vi "LS M81_Suslov.vi"(1 "Action":T6=enum."Identify", 2 "Parameters":variant) -> (6 "Output":variant, 7 "Stop":bool)   [LabVIEW 2021]
uses:
  Sub Controls/Instrument Actions.ctl
  Sub Controls/Public.ctl
  Sub Controls/Instrument Match.ctl
  SubVIs/M81 Sensor Options.ctl
  Sub Controls/Factory Reset.ctl
  Sub Controls/Scan Output.ctl
  Sub Controls/Instrument IDN.ctl
  Sub Controls/User Event Command.ctl
  <vilib>/Instr/_visa.llb/VISA GPIB Control REN Mode.ctl
panel:
  in  "DC_AC Measurements":enum32{"DC", "Total RMS", "AC Peak-to-Peak"}(radio)
  out "Instrument Name":string
  in  "Source Mode":T1(radio)=enum."DC"
  in  "Sensor Mode":enum32{"No Selection", "DC", "AC", "Lockin"}(radio)=enum."DC"
  in  "Slot #":enum32{"Slot 1", "Slot 2", "Slot 3"}(radio)
  in  "Source Parameters":enum32{"DC Offset", "Peak-to-Peak/2", "Both"}(radio)=enum."Peak-to-Peak/2"
  in  "Factory Reset":T2
  out "Channel Index":i32
  in  "Lockin Measurements: RMS":T3={"X"=TRUE, "X&Y"=FALSE, "R"=FALSE, "R & ϴ"=FALSE}
  out "Title":string="Lake Shore M-81 Modules"
  in  "VISA resource name":refnum<visa-resource-name>
  in  "Instruments":T4[](array[typedef])=[{"Model"="VS-10", "Manufacturer"="Lake Shore", "Term Character"="", "Wait Time (mS)"=0, "Wait for SRQ"=FALSE, "Type"=""}, {"Model"="BCS-10", "Manufacturer"="Lake Shore", "Term Character"="", "Wait Time (mS)"=0, "Wait for SRQ"=FALSE, "Type"=""}, {"Model"="VM-10", "Manufacturer"="Lake Shore", "Term Character"="", "Wait Time (mS)"=0, "Wait for SRQ"=FALSE, "Type"=""}, {"Model"="CM-10", "Manufacturer"="Lake Shore", "Term Character"="", "Wait Time (mS)"=0, "Wait for SRQ"=FALSE, "Type"=""}]
  out "Model":string
  in  "Address":u16(ring)
  in  "Public":T5
  out "Measurement":dbl[](array[numeric]) format="%^.3e"
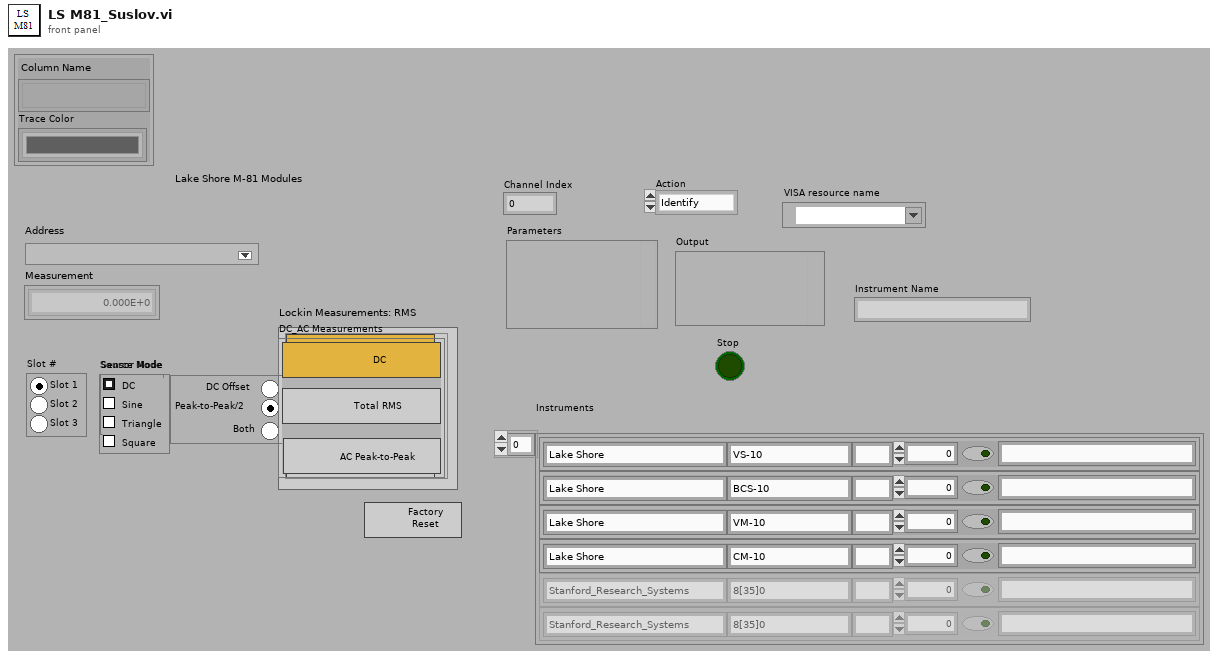
[diagram p1: front panel]
types:
  T1 = enum32{"No Selection", "DC", "Sine", "Triangle", "Square"}
  T2 = typedef "Factory Reset.ctl" = bool
  T3 = typedef "M81 Sensor Options.ctl" = cluster{"X":bool, "X&Y":bool, "R":bool, "R & ϴ":bool}
  T4 = typedef "Instrument Match.ctl" = cluster{"Model":string, "Manufacturer":string, "Term Character":string, "Wait Time (mS)":u32, "Wait for SRQ":bool, "Type":string}
  T5 = typedef "Public.ctl" = cluster{"Column Name":string[], "Trace Color":u32[]}
  T6 = typedef "Instrument Actions.ctl" = enum16{"Scan", "Identify", "New", "Configure", "Initialize", "Test", "Read", "Close"}
  T7 = typedef "Scan Output.ctl" = cluster{"Manufacturer":string, "Model":string, "Info":string, "Revision":string, "error out":errorcluster}
  T8 = typedef "Instrument IDN.ctl" = cluster{"VISA Address":string, "Status":u16, "Manufacturer":string, "Model":string, "Info":string, "Info 2":string, "Misc Data":variant}
  T9 = enum8{"Enabled", "Disabled", "Disabled and Grayed Out"}
  T10 = typedef "User Event Command.ctl" = enum32{"Stop Config"}
  T11 = typedef "VISA GPIB Control REN Mode.ctl" = u16
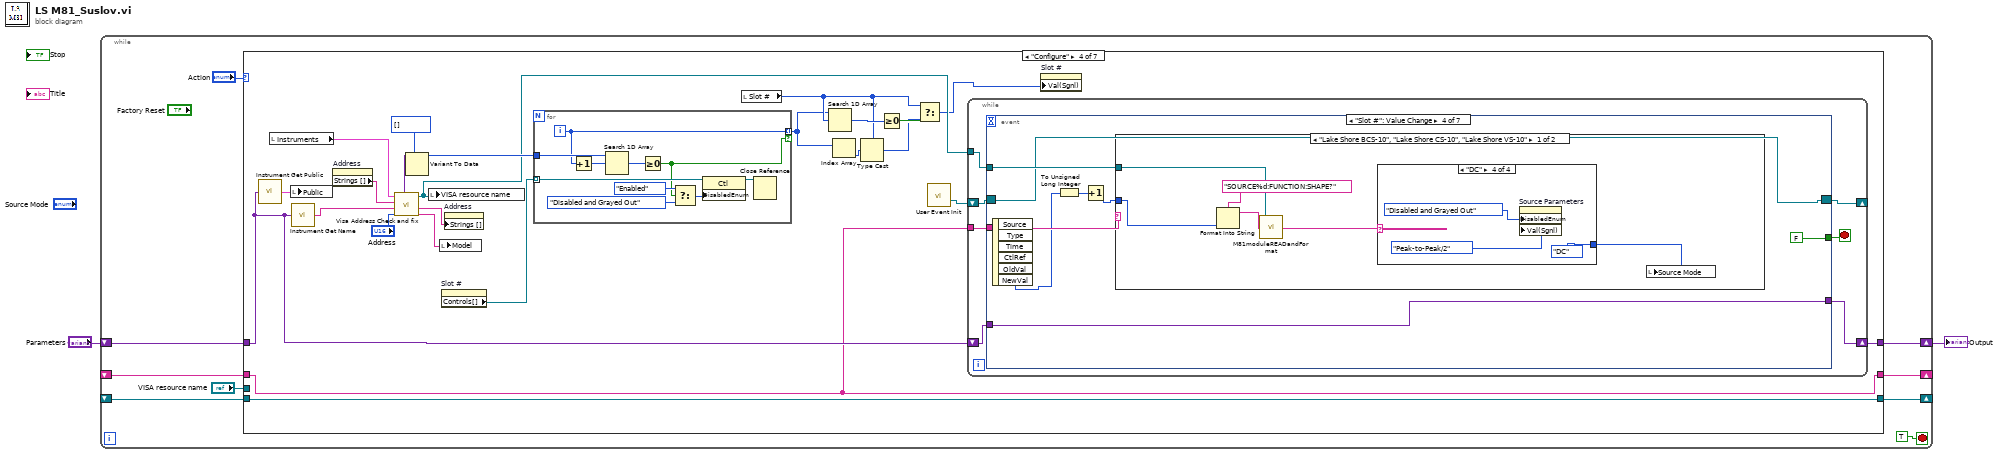
[diagram p0: block diagram]
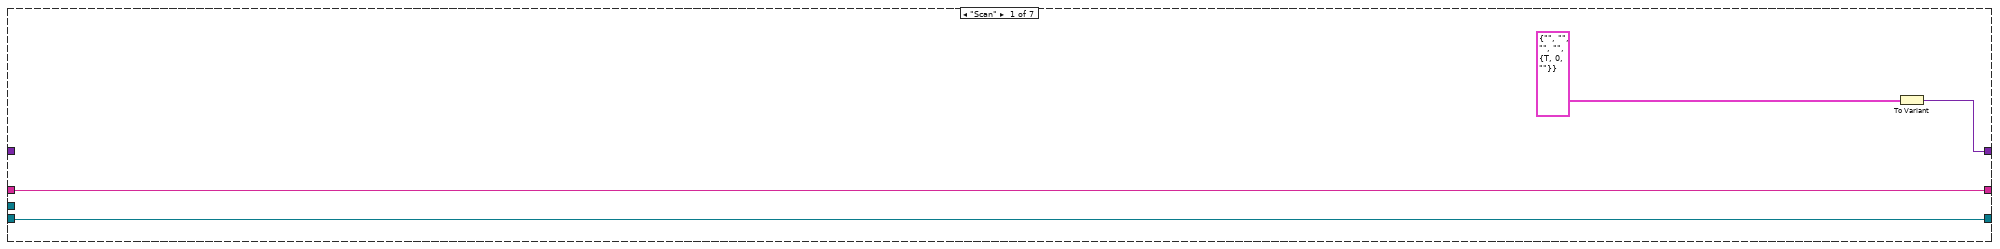
[diagram p2: hidden frame]
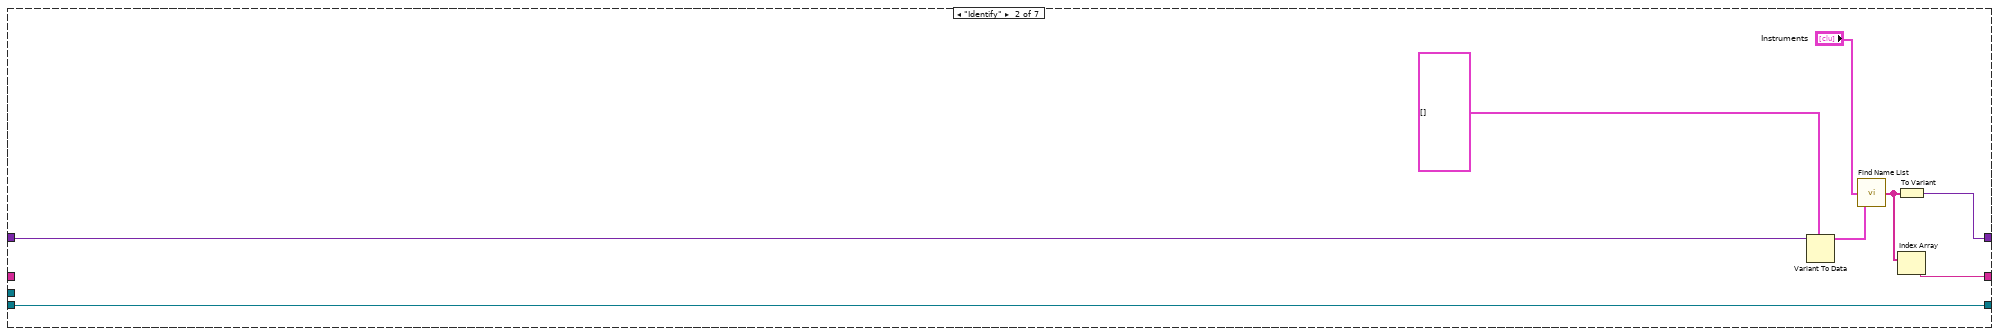
[diagram p3: hidden frame]
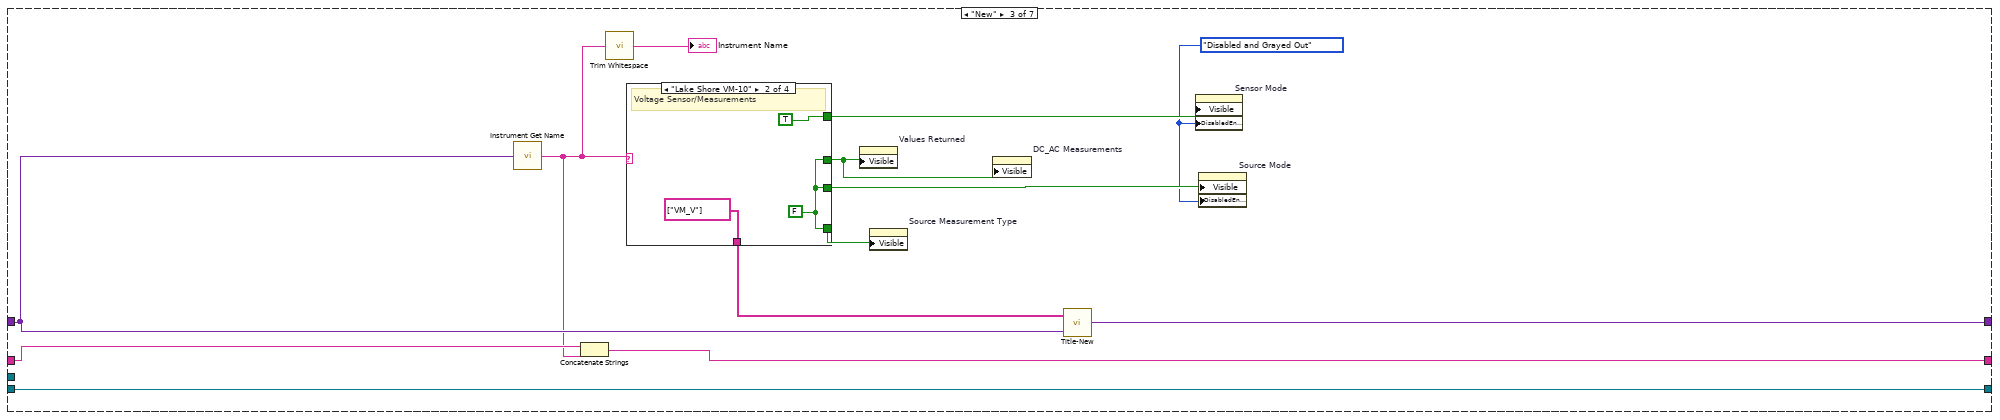
[diagram p4: hidden frame]
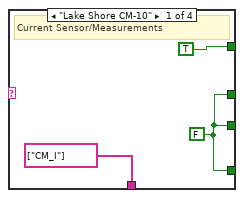
[diagram p5: hidden frame]
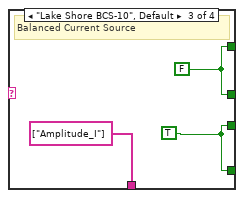
[diagram p6: hidden frame]
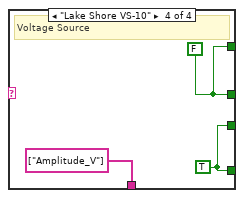
[diagram p7: hidden frame]
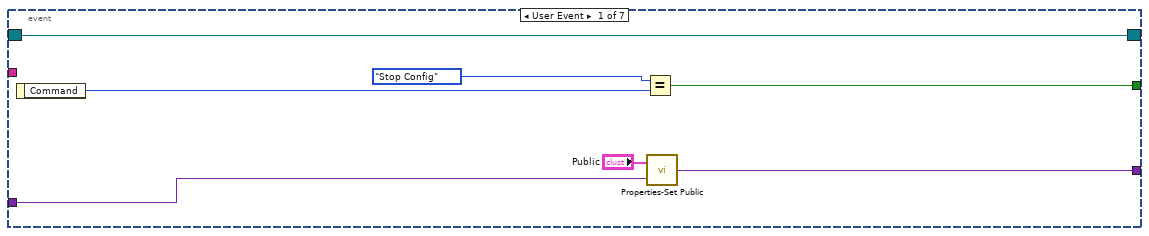
[diagram p8: hidden frame]
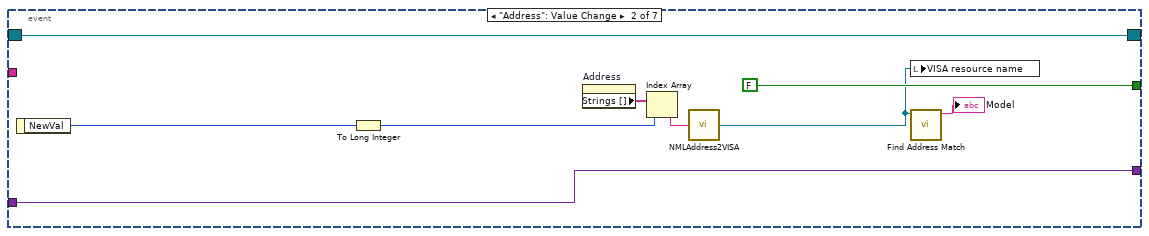
[diagram p9: hidden frame]
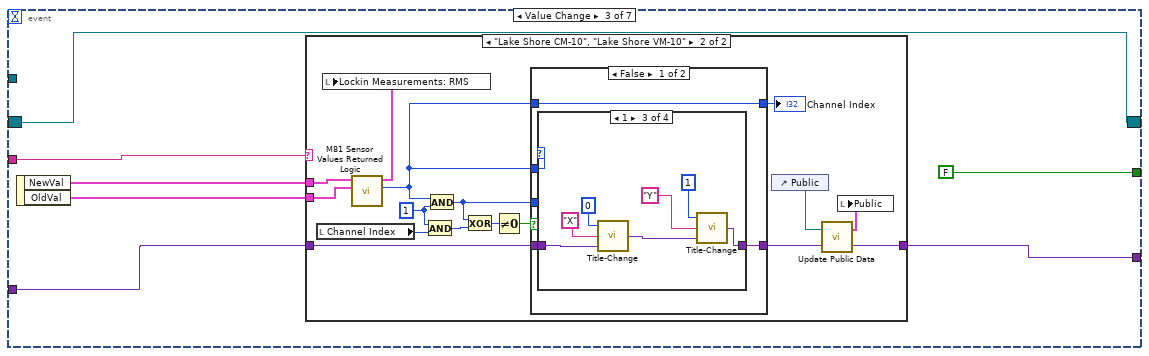
[diagram p10: hidden frame]
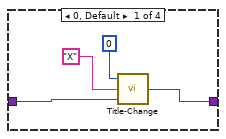
[diagram p12: hidden frame]
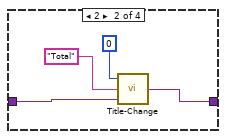
[diagram p13: hidden frame]
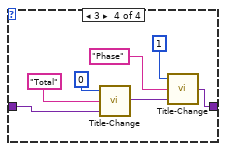
[diagram p14: hidden frame]
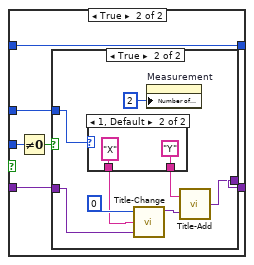
[diagram p15: hidden frame]
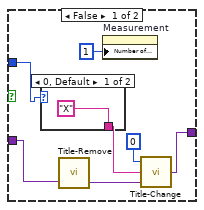
[diagram p16: hidden frame]
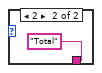
[diagram p17: hidden frame]
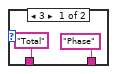
[diagram p18: hidden frame]
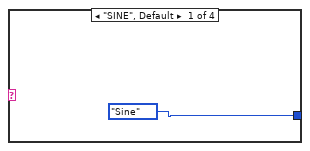
[diagram p19: hidden frame]
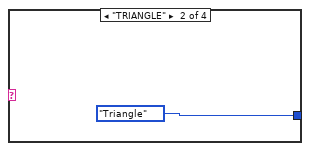
[diagram p20: hidden frame]
diagram:
  n1 = while {
    shift-right: [w10] -> _
    shift-left: _ -> [w9]
    shift-right: [w7] -> w1
    shift-left: "Parameters" -> [w8]
    shift-right: [w4] -> _
    shift-left: _ -> [w3]
    stop <- TRUE stop-if-true
    n2 = case shown="\"Configure\"" "Action" {
      tunnel: [w14 w23 w36 w72 w371 w382 refnum<visa-resource-name> refnum ("Open VISA Resource name")] -> w10
      tunnel: w9 -> [w14 w23 w36 w72 _ w381 w420]
      tunnel: w8 -> [_ w20 w34 w63 _ _ _]
      tunnel: [w13 w22 w35 w71 variant ("Variant") w389 variant ("Variant")] -> w7
      tunnel: "VISA resource name" -> [_ _ _ _ w373 _ _]
      tunnel: [w12 w16 w30 w52 w372 w388 w419] -> w4
      tunnel: w3 -> [w12 _ w31 w52 w372 w388 w419]
      frame "Scan" {
        n3 = To Variant(anything=T7 {"Manufacturer"="", "Model"="", "Info"="", "Revision"="", "error out"={"status"=TRUE, "code"=0, "source"=""}} ("Scan Output")) -> (Variant=w13:variant)
      }
      frame "Identify" {
        n4 = Variant To Data(type=T8[] [], Variant=w20) -> (data=w18:T8[])  [unwired: 1 in, 1 out]
        n5 = call "Find Name List.vi"("Bus Scan"=w18, "Instruments"="Instruments") -> ("Names"=w17:string[])  [unwired: 1 in]
        n6 = To Variant(anything=w17) -> (Variant=w22:variant)
        n7 = Index Array(array=w17) -> (element=w16:string)  [unwired: 1 in]
      }
      frame "New" {
        w25 = T9."Disabled and Grayed Out" ("Disabled")
        n8 = call "Instrument Get Name.vi"("Parameters"=w34) -> ("Type"=w26:string)
        n9 = Concatenate Strings(w31, w26) -> (w30:string)
        n10 = call <vilib>:"Trim Whitespace.vi"("string"=w26) -> ("trimmed string"=→"Instrument Name":string)  [unwired: 1 in]
        n11 = case shown="\"Lake Shore VM-10\"" w26 {
          tunnel: [w37 w40 w44 w47] -> w24
          tunnel: [w37 w40 w43 w46] -> w33
          tunnel: [string[] ["CM_I"] ("Array") string[] ["VM_V"] ("Array") string[] ["Amplitude_I"] ("Array") string[] ["Amplitude_V"] ("Array")] -> w32
          tunnel: [TRUE TRUE w44 w47] -> w29
          tunnel: [w37 w40 w43 w46] -> w28
          frame "Lake Shore CM-10" {
            w37 = FALSE
            # "Current Sensor/Measurements"
          }
          frame "Lake Shore VM-10" {
            w40 = FALSE
            # "Voltage Sensor/Measurements"
          }
          frame "Lake Shore BCS-10", Default {
            w43 = TRUE
            w44 = FALSE
            # "Balanced Current Source"
          }
          frame "Lake Shore VS-10" {
            w46 = TRUE
            w47 = FALSE
            # "Voltage Source"
          }
        }
        n12 = property on="Values Returned" class="Clust (strict)"("Visible"=w24) -> ()  [unwired: 2 in, 2 out]
        n13 = property on="Source Measurement Type" class="RadioBtnsControl (strict)"("Visible"=w33) -> ()  [unwired: 2 in, 2 out]
        n14 = property on="DC_AC Measurements" class="RadioBtnsControl (strict)"("Visible"=w24) -> ()  [unwired: 2 in, 2 out]
        n15 = call "Title-New.vi"("Parameters"=w34, "Array"=w32) -> ("Instrument Prop"=w35:variant)
        n16 = property on="Sensor Mode" class="RadioBtnsControl (strict)"("Visible"=w29, "DisabledEnum"=w25) -> ()  [unwired: 2 in, 2 out]
        n17 = property on="Source Mode" class="RadioBtnsControl (strict)"("Visible"=w28, "DisabledEnum"=w25) -> ()  [unwired: 2 in, 2 out]
      }
      frame "Configure" {
        n18 = call "Instrument Get Public.vi"("Variant"=w63) -> ("Public"=w70:T5)
        n19 = local read "Instruments"() -> (w62:T4[])
        n20 = local write "Public"(w70) -> ()
        n21 = call "Instrument Get Name.vi"("Parameters"=w63) -> ("Type"=w64:string)
        n22 = property on="Address" class="Ring (strict)"() -> ("Strings []"=w67:string[])  [unwired: 2 in, 2 out]
        n23 = call "Visa Address Check and fix.vi"("Instruments"=w62, "NML Addresses"=w67, "Name"=w64, "Address"="Address") -> ("Array"=w60:variant[], "VISA resource name"=w51:refnum<visa-resource-name>, "NML Addresses"=w66:string[], "Model"=w65:string)  [unwired: 3 out]
        n24 = Variant To Data(type=i32[] [], Variant=w60) -> (data=w59:i32[])  [unwired: 1 in, 1 out]
        n25 = local write "VISA resource name"(w51) -> ()
        n26 = local write "Model"(w65) -> ()
        n27 = property on="Slot #" class="RadioBtnsControl (strict)"() -> ("Controls[]"=w58:refnum<vi>[])  [unwired: 2 in, 2 out]
        n28 = property on="Address" class="Ring (strict)"("Strings []"=w66) -> ()  [unwired: 2 in, 2 out]
        n29 = for {
          tunnel: w58 -> [w80] mode=indexing
          tunnel: w59 -> [w82]
          tunnel: [w75] -> w50 mode=indexing if=w74
          i -> [w75]
          n30 = Increment(x=w75) -> (x+1=w73:i32)
          n31 = Search 1D Array(1D array=w82, element=w73) -> (index of element=w81:i32)  [unwired: 1 in]
          n32 = Greater Or Equal To 0?(x=w81) -> (x >= 0?=w74:bool)
          n33 = Select(t=T9."Enabled" ("Disabled"), s=w74, f=T9."Disabled and Grayed Out" ("Disabled")) -> (s? t:f=w77:T9)
          n34 = property class="Ctl"(reference=w80, "DisabledEnum"=w77) -> (reference out=w79:refnum<vi>)  [unwired: 1 in, 1 out]
          n35 = Close Reference(reference=w79) -> ()  [unwired: 1 in, 1 out]
        }
        n36 = local read "Slot #"() -> (w53:enum32{"Slot 1", "Slot 2", "Slot 3"})
        n37 = Search 1D Array(1D array=w50, element=w53) -> (index of element=w57:i32)  [unwired: 1 in]
        n38 = Index Array(array=w50) -> (element=w55:i32)  [unwired: 1 in]
        n39 = Type Cast(type=w53, x=w55) -> (*(type *) &x=w54:enum32{"Slot 1", "Slot 2", "Slot 3"})
        n40 = Greater Or Equal To 0?(x=w57) -> (x >= 0?=w56:bool)
        n41 = Select(t=w53, s=w56, f=w54) -> (s? t:f=w49:enum32{"Slot 1", "Slot 2", "Slot 3"})
        n42 = call "User Event Init.vi"() -> ("Event Registration Refnum"=w69:refnum<event-registration>)  [unwired: 14 in, 1 out]
        n43 = while {
          shift-right: [w89] -> w71
          shift-left: w63 -> [w88]
          shift-right: [w85] -> _
          shift-left: w69 -> [w86]
          tunnel: w52 -> [w84]
          tunnel: w51 -> [w83]
          stop <- w87 stop-if-true
          n44 = event shown="[3] \"Slot #\": Value Change" {
            selector: w86 -> [w90 w105 w111 w185 w228 w321 w368]
            dyn-events: [w90 w105 w111 w185 w228 w321 w368] -> w85
            timeout: _ -> [_ _ _ _ _ _ _]
            tunnel: [w92 FALSE FALSE FALSE FALSE FALSE FALSE] -> w87
            tunnel: w88 -> [w95 w99 w109 w189 w225 w319 w369]
            tunnel: [w96 w99 w110 w189 w223 w317 w369] -> w89
            tunnel: w84 -> [_ _ w106 w187 w224 w318 w366]
            tunnel: w83 -> [_ _ _ w190 _ _ _]
            event User Event {
              n45 = event-data() -> ("Command"=w94:T10)  [unwired: 1 in]
              n46 = Equal?(x=User_Event_Command."Stop Config", y=w94) -> (x = y?=w92:bool)
              n47 = call "Properties-Set Public.vi"("Variant"=w95, "New Public"="Public") -> ("Variant 2"=w96:variant)
            }
            event "Address": Value Change {
              n48 = event-data() -> ("NewVal"=w103:u16)  [unwired: 1 in]
              n49 = To Long Integer(number=w103) -> (32bit integer=w97:i32)
              n50 = property on="Address" class="Ring (strict)"() -> ("Strings []"=w102:string[])  [unwired: 2 in, 2 out]
              n51 = Index Array(array=w102, index=w97) -> (element=w101:string)
              n52 = call "NMLAddress2VISA.vi"("NML Address"=w101) -> ("VISA resource name"=w98:refnum<visa-resource-name>)
              n53 = local write "VISA resource name"(w98) -> ()
              n54 = call "Find Address Match.vi"("VISA resource name"=w98) -> ("Model"=→"Model":string)  [unwired: 3 in, 3 out]
            }
            event Value Change {
              n55 = event-data() -> ("NewVal"=w108:T3, "OldVal"=w107:T3)  [unwired: 1 in]
              n56 = case shown="\"Lake Shore CM-10\", \"Lake Shore VM-10\"" w106 {
                tunnel: [w113 w127] -> w110
                tunnel: w109 -> [w113 w125]
                tunnel: w108 -> [_ w124]
                tunnel: w107 -> [_ w123]
                frame "False", Default {
                }
                frame "Lake Shore CM-10", "Lake Shore VM-10" {
                  w118 = 1 ("y")
                  n57 = local read "Channel Index"() -> (w121:i32)
                  n58 = call "M81 Sensor Values Returned Logic.vi"("Old Channels"=w123, "New Channels"=w124) -> ("index of element"=w114:i32, "Channels Out"=w122:T3)  [unwired: 8 in]
                  n59 = local write "Lockin Measurements: RMS"(w122) -> ()
                  n60 = And(x=w118, y=w121) -> (x .and. y?=w119:i32)
                  n61 = And(x=w114, y=w118) -> (x .and. y?=w116:i32)
                  n62 = Exclusive Or(1:w119, 2:w116) -> (0:w120:i32)
                  n63 = Not Equal To 0?(x=w120) -> (x != 0?=w117:bool)
                  n64 = case shown="False" w117 {
                    tunnel: [w130 w161] -> w129
                    tunnel: w125 -> [w131 w160]
                    tunnel: w116 -> [_ w159]
                    tunnel: w114 -> [w133 w157]
                    tunnel: [w133 w157] -> w115
                    tunnel: w114 -> [w132 w156]
                    frame False {
                      n65 = case shown="1" w132 {
                        tunnel: w131 -> [w136 w140 w146 w153]
                        tunnel: [w135 w139 w142 w149] -> w130
                        frame 0, Default {
                          n66 = call "Title-Change.vi"("Parameters"=w136, "New Title"="X", "Index"=0) -> ("Variant"=w135:variant)
                        }
                        frame 2 {
                          n67 = call "Title-Change.vi"("Parameters"=w140, "New Title"="Total", "Index"=0) -> ("Variant"=w139:variant)
                        }
                        frame 1 {
                          n68 = call "Title-Change.vi"("Parameters"=w146, "New Title"="X", "Index"=0) -> ("Variant"=w143:variant)
                          n69 = call "Title-Change.vi"("Parameters"=w143, "New Title"="Y", "Index"=1) -> ("Variant"=w142:variant)
                        }
                        frame 3 {
                          n70 = call "Title-Change.vi"("Parameters"=w153, "New Title"="Total", "Index"=0) -> ("Variant"=w150:variant)
                          n71 = call "Title-Change.vi"("Parameters"=w150, "New Title"="Phase", "Index"=1) -> ("Variant"=w149:variant)
                        }
                      }
                    }
                    frame True {
                      n72 = Not Equal To 0?(x=w159) -> (x != 0?=w158:bool)
                      n73 = case shown="True" w158 {
                        tunnel: w160 -> [w167 w173]
                        tunnel: [w163 w178] -> w161
                        tunnel: w156 -> [w162 w175]
                        frame False {
                          n74 = case shown="0, Default" w162 {
                            tunnel: ["X" ("Title") "Total" ("Title")] -> w166
                            frame 0, Default {
                            }
                            frame 2 {
                            }
                          }
                          n75 = call "Title-Remove.vi"("Parameters"=w167) -> ("Variant"=w164:variant)  [unwired: 1 in]
                          n76 = property on="Measurement" class="Arr (strict)"("Number of Columns"=u32 1) -> ()  [unwired: 2 in, 2 out]
                          n77 = call "Title-Change.vi"("Parameters"=w164, "New Title"=w166, "Index"=0) -> ("Variant"=w163:variant)
                        }
                        frame True {
                          n78 = case shown="1, Default" w175 {
                            tunnel: ["Phase" ("String") "Y" ("String")] -> w177
                            tunnel: ["Total" ("String") "X" ("String")] -> w172
                            frame 3 {
                            }
                            frame 1, Default {
                            }
                          }
                          n79 = call "Title-Change.vi"("Parameters"=w173, "New Title"=w172, "Index"=0) -> ("Variant"=w171:variant)
                          n80 = property on="Measurement" class="Arr (strict)"("Number of Columns"=u32 2) -> ()  [unwired: 2 in, 2 out]
                          n81 = call "Title-Add.vi"("Parameters"=w171, "String"=w177) -> ("Variant"=w178:variant)
                        }
                      }
                    }
                  }
                  "Channel Index" <- w115
                  n82 = control-ref of="Public"() -> (w128:refnum<vi>)
                  n83 = call "Update Public Data.vi"("Variant In"=w129, "Public 2"=w128) -> ("Variant Out"=w127:variant, "Public"=w126:T5)
                  n84 = local write "Public"(w126) -> ()
                }
              }
            }
            event "Slot #": Value Change {
              n85 = event-data() -> ("NewVal"=w183:enum32{"Slot 1", "Slot 2", "Slot 3"})  [unwired: 1 in, 5 out]
              n86 = To Unsigned Long Integer(number=w183) -> (unsigned 32bit integer=w184:u32)
              n87 = Increment(x=w184) -> (x+1=w186:u32)
              n88 = case shown="\"Lake Shore BCS-10\", \"Lake Shore CS-10\", \"Lake Shore VS-10\"" w187 {
                tunnel: w186 -> [w194 w208]
                tunnel: w190 -> [w193 w207]
                frame "Lake Shore BCS-10", "Lake Shore CS-10", "Lake Shore VS-10" {
                  n89 = Format Into String(format string="SOURCE%d:FUNCTION:SHAPE?" ("write buffer (\"\")"), w194) -> (resulting string=w195:string)  [unwired: 2 in, 1 out]
                  n90 = call "M81moduleREADandFormat.vi"("Command"=w195, "VISA resource name"=w193) -> ("result string"=w191:string)  [unwired: 1 in, 2 out]
                  n91 = case shown="\"DC\"" w191 {
                    tunnel: [T1."Sine" ("Source Mode") T1."Triangle" ("Source Mode") T1."Square" ("Source Mode") T1."DC" ("Source Mode")] -> w192
                    frame "SINE", Default {
                    }
                    frame "TRIANGLE" {
                    }
                    frame "SQUARE" {
                    }
                    frame "DC" {
                      n92 = property on="Source Parameters" class="RadioBtnsControl (strict)"("DisabledEnum"=T9."Disabled and Grayed Out" ("Disabled"), "Val(Sgnl)"=enum32{"DC Offset", "Peak-to-Peak/2", "Both"}."Peak-to-Peak/2" ("Value (Signaling)")) -> ()  [unwired: 2 in, 2 out]
                    }
                  }
                  n93 = local write "Source Mode"(w192) -> ()
                }
                frame " Lake Shore VM-10", "Lake Shore CM-10", Default {
                  n94 = Format Into String(format string="SENSE%d:MODE?" ("write buffer (\"\")"), w208) -> (resulting string=w209:string)  [unwired: 2 in, 1 out]
                  n95 = call "M81moduleREADandFormat.vi"("Command"=w209, "VISA resource name"=w207) -> ("result string"=w206:string)  [unwired: 1 in, 2 out]
                  n96 = case shown="\"AC\", Default" w206 {
                    tunnel: [enum32{"No Selection", "DC", "AC", "Lockin"}."AC" ("Sensor Mode") enum32{"No Selection", "DC", "AC", "Lockin"}."Lockin" ("Sensor Mode") enum32{"No Selection", "DC", "AC", "Lockin"}."DC" ("Sensor Mode")] -> w205
                    tunnel: [FALSE ("Visible") TRUE FALSE ("Visible")] -> w204
                    tunnel: [TRUE FALSE ("Visible") TRUE] -> w203
                    frame "AC", Default {
                      n97 = property on="DC_AC Measurements" class="RadioBtnsControl (strict)"("DisabledEnum"=T9."Enabled" ("Disabled")) -> ()  [unwired: 2 in, 2 out]
                    }
                    frame "LIA" {
                    }
                    frame "DC" {
                      n98 = property on="DC_AC Measurements" class="RadioBtnsControl (strict)"("DisabledEnum"=T9."Disabled and Grayed Out" ("Disabled"), "Val(Sgnl)"=enum32{"DC", "Total RMS", "AC Peak-to-Peak"}."DC" ("DC_AC Measurements")) -> ()  [unwired: 2 in, 2 out]
                    }
                  }
                  n99 = property on="Values Returned: RMS" class="Clust (strict)"("Visible"=w204) -> ()  [unwired: 2 in, 2 out]
                  n100 = local write "Sensor Mode"(w205) -> ()
                  n101 = property on="DC_AC Measurements" class="RadioBtnsControl (strict)"("Visible"=w203) -> ()  [unwired: 2 in, 2 out]
                }
              }
            }
            event "Source Parameters": Value Change {
              # "VS-10\nshould be tested"
              n102 = event-data() -> ("OldVal"=w226:enum32{"DC Offset", "Peak-to-Peak/2", "Both"}, "NewVal"=w227:enum32{"DC Offset", "Peak-to-Peak/2", "Both"})  [unwired: 1 in]
              n103 = case shown="\"Lake Shore VS-10\"" w224 {
                tunnel: w227 -> [_ w237 w280]
                tunnel: w226 -> [_ w236 w279]
                tunnel: w225 -> [w230 w235 w278]
                tunnel: [w230 w231 w274] -> w223
                frame "False", Default {
                }
                frame "Lake Shore VS-10" {
                  n104 = case shown="\"DC Offset\", \"Peak-to-Peak/2\", Default" w236 {
                    tunnel: [w238 w260] -> w232
                    tunnel: w235 -> [w239 w259]
                    tunnel: w237 -> [w240 w258]
                    frame "DC Offset", "Peak-to-Peak/2", Default {
                      n105 = case shown="\"Both\"" w240 {
                        tunnel: w239 -> [w243 w248 w255]
                        tunnel: [w242 w251 w254] -> w238
                        frame "DC Offset", Default {
                          n106 = property on="Measurement" class="Arr (strict)"("Number of Columns"=u32 1) -> ()  [unwired: 2 in, 2 out]
                          n107 = call "Title-Change.vi"("Parameters"=w243, "New Title"="Offset_V" ("Title"), "Index"=0) -> ("Variant"=w242:variant)
                        }
                        frame "Both" {
                          n108 = property on="Measurement" class="Arr (strict)"("Number of Columns"=u32 2) -> ()  [unwired: 2 in, 2 out]
                          n109 = call "Title-Change.vi"("Parameters"=w248, "New Title"="Offset_V" ("Title"), "Index"=0) -> ("Variant"=w247:variant)
                          n110 = call "Title-Add.vi"("Parameters"=w247, "String"="Amplitude_V") -> ("Variant"=w251:variant)
                        }
                        frame "Peak-to-Peak/2" {
                          n111 = property on="Measurement" class="Arr (strict)"("Number of Columns"=u32 1) -> ()  [unwired: 2 in, 2 out]
                          n112 = call "Title-Change.vi"("Parameters"=w255, "New Title"="Amplitude_V" ("Title"), "Index"=0) -> ("Variant"=w254:variant)
                        }
                      }
                    }
                    frame "Both" {
                      n113 = case shown="\"DC Offset\"" w258 {
                        tunnel: w259 -> [w266 w272 w273]
                        tunnel: [w261 w267 w273] -> w260
                        frame "DC Offset" {
                          n114 = property on="Measurement" class="Arr (strict)"("Number of Columns"=u32 1) -> ()  [unwired: 2 in, 2 out]
                          n115 = call "Title-Remove.vi"("Parameters"=w266) -> ("Variant"=w262:variant)  [unwired: 1 in]
                          n116 = call "Title-Change.vi"("Parameters"=w262, "New Title"="Offset_V" ("Title"), "Index"=0) -> ("Variant"=w261:variant)
                        }
                        frame "Peak-to-Peak/2" {
                          n117 = property on="Measurement" class="Arr (strict)"("Number of Columns"=u32 1) -> ()  [unwired: 2 in, 2 out]
                          n118 = call "Title-Remove.vi"("Parameters"=w272) -> ("Variant"=w268:variant)  [unwired: 1 in]
                          n119 = call "Title-Change.vi"("Parameters"=w268, "New Title"="Amplitude_V" ("Title"), "Index"=0) -> ("Variant"=w267:variant)
                        }
                        frame "Both" {
                        }
                      }
                    }
                  }
                  n120 = control-ref of="Public"() -> (w233:refnum<vi>)
                  n121 = call "Update Public Data.vi"("Variant In"=w232, "Public 2"=w233) -> ("Variant Out"=w231:variant, "Public"=w234:T5)
                  n122 = local write "Public"(w234) -> ()
                }
                frame "Lake Shore BCS-10" {
                  n123 = case shown="\"DC Offset\", \"Peak-to-Peak/2\", Default" w279 {
                    tunnel: [w281 w303] -> w275
                    tunnel: w278 -> [w282 w302]
                    tunnel: w280 -> [w283 w301]
                    frame "DC Offset", "Peak-to-Peak/2", Default {
                      n124 = case shown="\"Both\"" w283 {
                        tunnel: w282 -> [w286 w291 w298]
                        tunnel: [w285 w294 w297] -> w281
                        frame "DC Offset", Default {
                          n125 = property on="Measurement" class="Arr (strict)"("Number of Columns"=u32 1) -> ()  [unwired: 2 in, 2 out]
                          n126 = call "Title-Change.vi"("Parameters"=w286, "New Title"="Offset_I" ("Title"), "Index"=0) -> ("Variant"=w285:variant)
                        }
                        frame "Both" {
                          n127 = property on="Measurement" class="Arr (strict)"("Number of Columns"=u32 2) -> ()  [unwired: 2 in, 2 out]
                          n128 = call "Title-Change.vi"("Parameters"=w291, "New Title"="Offset_I" ("Title"), "Index"=0) -> ("Variant"=w290:variant)
                          n129 = call "Title-Add.vi"("Parameters"=w290, "String"="Amplitude_I") -> ("Variant"=w294:variant)
                        }
                        frame "Peak-to-Peak/2" {
                          n130 = property on="Measurement" class="Arr (strict)"("Number of Columns"=u32 1) -> ()  [unwired: 2 in, 2 out]
                          n131 = call "Title-Change.vi"("Parameters"=w298, "New Title"="Amplitude_I" ("Title"), "Index"=0) -> ("Variant"=w297:variant)
                        }
                      }
                    }
                    frame "Both" {
                      n132 = case shown="\"DC Offset\"" w301 {
                        tunnel: w302 -> [w309 w315 w316]
                        tunnel: [w304 w310 w316] -> w303
                        frame "DC Offset" {
                          n133 = property on="Measurement" class="Arr (strict)"("Number of Columns"=u32 1) -> ()  [unwired: 2 in, 2 out]
                          n134 = call "Title-Remove.vi"("Parameters"=w309) -> ("Variant"=w305:variant)  [unwired: 1 in]
                          n135 = call "Title-Change.vi"("Parameters"=w305, "New Title"="Offset_V" ("Title"), "Index"=0) -> ("Variant"=w304:variant)
                        }
                        frame "Peak-to-Peak/2" {
                          n136 = property on="Measurement" class="Arr (strict)"("Number of Columns"=u32 1) -> ()  [unwired: 2 in, 2 out]
                          n137 = call "Title-Remove.vi"("Parameters"=w315) -> ("Variant"=w311:variant)  [unwired: 1 in]
                          n138 = call "Title-Change.vi"("Parameters"=w311, "New Title"="Amplitude_V" ("Title"), "Index"=0) -> ("Variant"=w310:variant)
                        }
                        frame "Both" {
                        }
                      }
                    }
                  }
                  n139 = control-ref of="Public"() -> (w276:refnum<vi>)
                  n140 = call "Update Public Data.vi"("Variant In"=w275, "Public 2"=w276) -> ("Variant Out"=w274:variant, "Public"=w277:T5)
                  n141 = local write "Public"(w277) -> ()
                }
              }
            }
            event "DC_AC Measurements": Value Change {
              # "VS-10\nshould be tested"
              n142 = event-data() -> ("NewVal"=w320:enum32{"DC", "Total RMS", "AC Peak-to-Peak"})  [unwired: 1 in, 1 out]
              n143 = case shown="\"Lake Shore CM-10\"" w318 {
                tunnel: w320 -> [_ w329 w350]
                tunnel: w319 -> [w323 w328 w349]
                tunnel: [w323 w324 w345] -> w317
                frame "False", Default {
                }
                frame "Lake Shore VM-10" {
                  n144 = case shown="\"Total RMS\"" w329 {
                    tunnel: w328 -> [w332 w337 w342]
                    tunnel: [w331 w335 w341] -> w325
                    frame "DC", Default {
                      n145 = property on="Measurement" class="Arr (strict)"("Number of Columns"=u32 1) -> ()  [unwired: 2 in, 2 out]
                      n146 = call "Title-Change.vi"("Parameters"=w332, "New Title"="DC_V" ("Title"), "Index"=0) -> ("Variant"=w331:variant)
                    }
                    frame "AC Peak-to-Peak" {
                      n147 = property on="Measurement" class="Arr (strict)"("Number of Columns"=u32 1) -> ()  [unwired: 2 in, 2 out]
                      n148 = call "Title-Change.vi"("Parameters"=w337, "New Title"="ACptp_V" ("Title"), "Index"=0) -> ("Variant"=w335:variant)
                    }
                    frame "Total RMS" {
                      n149 = property on="Measurement" class="Arr (strict)"("Number of Columns"=u32 1) -> ()  [unwired: 2 in, 2 out]
                      n150 = call "Title-Change.vi"("Parameters"=w342, "New Title"="RMS_V" ("Title"), "Index"=0) -> ("Variant"=w341:variant)
                    }
                  }
                  n151 = control-ref of="Public"() -> (w326:refnum<vi>)
                  n152 = call "Update Public Data.vi"("Variant In"=w325, "Public 2"=w326) -> ("Variant Out"=w324:variant, "Public"=w327:T5)
                  n153 = local write "Public"(w327) -> ()
                }
                frame "Lake Shore CM-10" {
                  n154 = case shown="\"DC\", Default" w350 {
                    tunnel: w349 -> [w353 w358 w363]
                    tunnel: [w352 w356 w362] -> w346
                    frame "DC", Default {
                      n155 = property on="Measurement" class="Arr (strict)"("Number of Columns"=u32 1) -> ()  [unwired: 2 in, 2 out]
                      n156 = call "Title-Change.vi"("Parameters"=w353, "New Title"="DC_I" ("Title"), "Index"=0) -> ("Variant"=w352:variant)
                    }
                    frame "AC Peak-to-Peak" {
                      n157 = property on="Measurement" class="Arr (strict)"("Number of Columns"=u32 1) -> ()  [unwired: 2 in, 2 out]
                      n158 = call "Title-Change.vi"("Parameters"=w358, "New Title"="ACptp_I" ("Title"), "Index"=0) -> ("Variant"=w356:variant)
                    }
                    frame "Total RMS" {
                      n159 = property on="Measurement" class="Arr (strict)"("Number of Columns"=u32 1) -> ()  [unwired: 2 in, 2 out]
                      n160 = call "Title-Change.vi"("Parameters"=w363, "New Title"="RMS_I" ("Title"), "Index"=0) -> ("Variant"=w362:variant)
                    }
                  }
                  n161 = control-ref of="Public"() -> (w347:refnum<vi>)
                  n162 = call "Update Public Data.vi"("Variant In"=w346, "Public 2"=w347) -> ("Variant Out"=w345:variant, "Public"=w348:T5)
                  n163 = local write "Public"(w348) -> ()
                }
              }
            }
            event Value Change {
              n164 = event-data() -> ()  [unwired: 1 in, 1 out]
              n165 = call "Instrument Single Command.vi"("Reset Command"="RST", "VISA Name"=w366) -> ()  [unwired: 9 in, 1 out]
            }
          }
        }
        n166 = property on="Slot #" class="RadioBtnsControl (strict)"("Val(Sgnl)"=w49) -> ()  [unwired: 2 in, 2 out]
      }
      frame "Initialize" {
        w377 = T11 1 items=["Deassert REN", "Assert REN", "Go To Local; Deassert REN ", "Assert REN; Address Device", "Local Lockout (Addressed Devices)", "Local Lockout (This Device)", "Go To Local"] ("Mode")
        n167 = VISA Open(duplicate session (F)=TRUE, VISA resource name=w373) -> (VISA resource name=w375:refnum<visa-resource-name>, error out=w376:errorcluster)  [unwired: 3 in]
        n168 = VISA GPIB Control REN(8:w376, 10:w377, 11:w375) -> (3:w371:refnum<visa-resource-name>)  [unwired: 1 out]
      }
      frame "Test", "Read" {
        # "...the amplitude {command} sets the peak level of the excitation waveform  (p21)"
        # "Case \"Lake Shore VS-10\" should be tested when a module is available"
        n169 = case shown="\"Lake Shore BCS-10\", Default" w388 {
          tunnel: "Source Parameters" -> [w391 w396 _]
          tunnel: "Lockin Measurements: RMS" -> [_ _ w403]
          tunnel: "Sensor Mode" -> [_ _ w402]
          tunnel: "DC_AC Measurements" -> [_ _ w401]
          tunnel: [w390 w395 w400] -> w379
          frame "Lake Shore BCS-10", Default {
            n170 = case shown="\"Peak-to-Peak/2\", Default" w391 {
              tunnel: ["SOURCE%d:CURRENT:OFFSET?" ("format string") "SOURCE%d:CURRENT?" ("format string") "SOURCE%d:CURRENT:OFFSET?; CURRENT?" ("format string")] -> w390
              frame "DC Offset" {
                (unwired) "SOURCE%d:CURRENT:LEVEL:OFFSET?" ("format string")
              }
              frame "Peak-to-Peak/2", Default {
                (unwired) "SOURCE%d:CURRENT:LEVEL:AMPLITUDE?" ("format string")
              }
              frame "Both" {
                (unwired) "SOURCE%d:CURRENT:LEVEL:OFFSET?" ("format string")
                (unwired) "SOURCE%d:CURRENT:LEVEL:AMPLITUDE?" ("format string")
              }
            }
          }
          frame "Lake Shore VS-10" {
            n171 = case shown="\"Both\"" w396 {
              tunnel: ["SOURCE%d:VOLTAGE:OFFSET?" ("format string") "SOURCE%d:VOLTAGE?" ("format string") "SOURCE%d:VOLTAGE:OFFSET?; VOLTAGE?" ("format string")] -> w395
              frame "DC Offset" {
                (unwired) "SOURCE%d:VOLTAGE:LEVEL:OFFSET?" ("format string")
              }
              frame "Peak-to-Peak/2", Default {
                (unwired) "SOURCE%d:VOLTAGE:LEVEL:AMPLITUDE?" ("format string")
              }
              frame "Both" {
                (unwired) "SOURCE%d:VOLTAGE:LEVEL:OFFSET?" ("format string")
                (unwired) "SOURCE%d:VOLTAGE:LEVEL:AMPLITUDE?" ("format string")
                (unwired) "SOURCE%d:VOLTAGE?" ("format string")
              }
            }
          }
          frame "Lake Shore CM-10", "Lake Shore VM-10" {
            n172 = case shown="\"DC\", Default" w402 {
              tunnel: w403 -> [_ _ w414]
              tunnel: w401 -> [_ w406 _]
              tunnel: ["FETCH:SENSE%D:DC?" ("format string") w405 w410] -> w400
              frame "DC", Default {
                # "Mode: DC/AC/Lockin"
              }
              frame "AC" {
                # "Mode: DC/AC/Lockin"
                n173 = case shown="\"Total RMS\"" w406 {
                  tunnel: ["FETCH:SENSE%d:DC?" ("format string") "FETCH:SENSE%d:RMS?" ("format string") "FETCH:SENSE%D:PTPEAK?" ("format string")] -> w405
                  frame "DC", Default {
                    # "DC indication"
                  }
                  frame "Total RMS" {
                    # "including ac and dc"
                  }
                  frame "AC Peak-to-Peak" {
                  }
                }
              }
              frame "Lockin" {
                # "Mode: DC/AC/Lockin"
                n174 = Cluster To Array(cluster=w414) -> (array=w412:bool[])
                n175 = Search 1D Array(1D array=w412, element=TRUE) -> (index of element=w411:i32)  [unwired: 1 in]
                n176 = case shown="2" w411 {
                  tunnel: ["FETCH:SENSE%D:LIA:X?" ("format string") "FETCH:SENSE%D:LIA:X?;Y?" ("format string") "FETCH:SENSE%D:LIA:R?" ("format string") "FETCH:SENSE%D:LIA:R?;THETA?" ("format string")] -> w410
                  frame 0, Default {
                    # "X"
                  }
                  frame 1 {
                    # "X & Y"
                  }
                  frame 2 {
                    # "SQRT(X^2+Y^2)"
                  }
                  frame 3 {
                    # "SQRT(X^2+Y^2)  & Theta"
                  }
                }
              }
            }
          }
        }
        n177 = call "M81 Read Values_Suslov.vi"("Slot"="Slot #", "Command string"=w379, "VISA resource name"=w381) -> ("Resistance"=w383:dbl[], "VISA resource name"=w382:refnum<visa-resource-name>)  [unwired: 7 in]
        "Measurement" <- w383
        n178 = To Variant(anything=w383) -> (Variant=w389:variant)
      }
      frame "Close" {
        w424 = T11 2 items=["Deassert REN", "Assert REN", "Go To Local; Deassert REN ", "Assert REN; Address Device", "Local Lockout (Addressed Devices)", "Local Lockout (This Device)", "Go To Local"] ("Mode")
        n179 = VISA GPIB Control REN(10:w424, 11:w420) -> (0:w423:errorcluster, 3:w422:refnum<visa-resource-name>)  [unwired: 1 in]
        n180 = VISA Close(VISA resource name=w422, error in (no error)=w423) -> ()  [unwired: 1 out]
      }
    }
  }
  "Output" <- w1
